vi "script - Copy.vi"() -> ()   [LabVIEW 2021]
panel:
  out "VI Name 2":string
  out "Application:All VIs In Memory 2":string[](array[string])
  out "VI Name":string
  out "appended array":errorcluster[](array[cluster])
  out "Application:All VIs In Memory":string[](array[string])
  out "error out":errorcluster
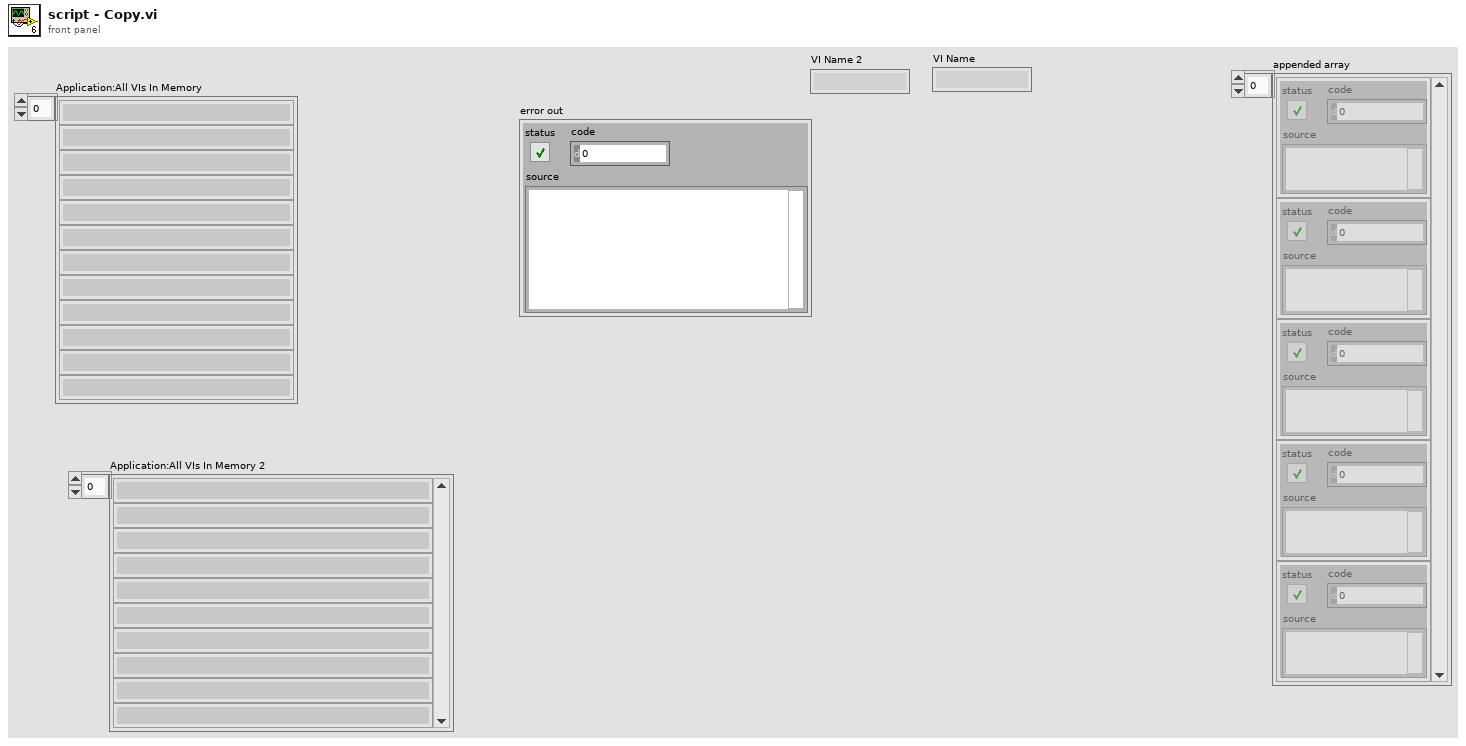
[diagram p1: front panel]
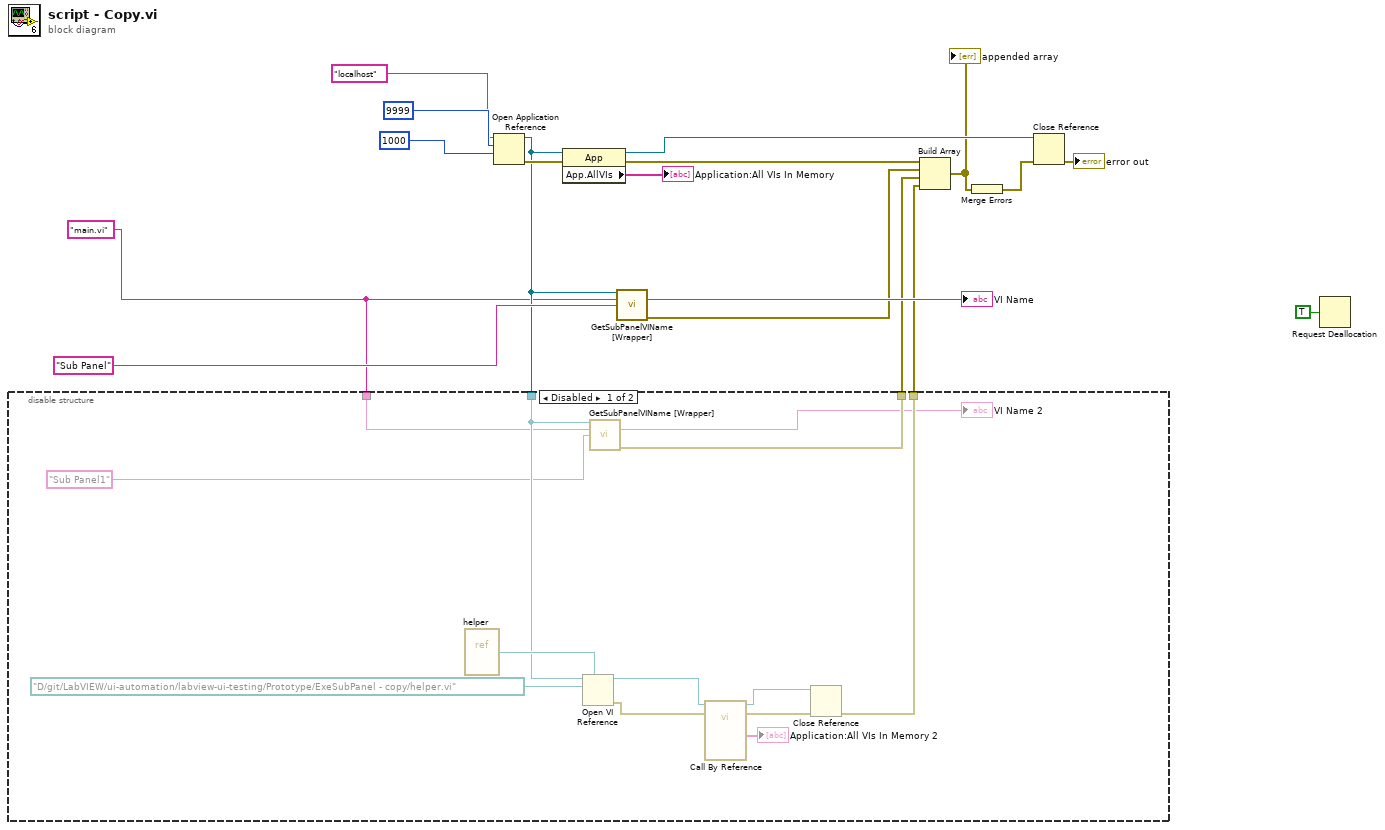
[diagram p0: block diagram]
diagram:
  w5 = "main.vi" ("y")
  n1 = Open Application Reference(9:1000 ("timeout ms (60000)"), 10:u16 9999 ("port number or service name (3363)"), 11:"localhost" ("machine name (\"\":  open local reference)")) -> (0:w17:errorcluster, 3:w6:refnum<vi>)  [unwired: 1 in]
  n2 = disable-structure shown="Disabled" {
    disable-tunnel: [w24 _] -> w8
    disable-tunnel: w6 -> [w23 _]
    disable-tunnel: w5 -> [w22 _]
    disable-tunnel: [w21 _] -> w4
    frame Disabled {
      n3 = vi-ref "helper.vi"() -> (w30:refnum<vi>)
      n4 = Open VI Reference(type specifier VI Refnum (for type only)=w30, application reference (local)=w23, vi path=path "D:/git/LabVIEW/ui-automation/labview-ui-testing/Prototype/ExeSubPanel - copy/helper.vi") -> (vi reference=w29:refnum<vi>, error out=w28:errorcluster)  [unwired: 3 in]
      n5 = call "GetSubPanelVIName [Wrapper].vi"("Application in"=w23, "VI Name"=w22, "SubPanel Label"="Sub Panel1" ("y")) -> ("VI Name"=→"VI Name 2":string, "error out"=w21:errorcluster)  [unwired: 10 in, 1 out]
      n6 = call-by-ref "?"(reference=w29, error in=w28) -> (reference out=w26:refnum<vi>, error out=w27:errorcluster, "Application:All VIs In Memory"=→"Application:All VIs In Memory 2":string[])  [unwired: 10 in, 1 out]
      n7 = Close Reference(reference=w26, error in (no error)=w27) -> (error out=w24:errorcluster)
    }
    frame Enabled {
    }
  }
  n8 = property class="App"(reference=w6, error in=w17) -> (reference out=w16:refnum<vi>, error out=w11:errorcluster, "App.AllVIs"=→"Application:All VIs In Memory":string[])
  n9 = call "GetSubPanelVIName [Wrapper].vi"("Application in"=w6, "VI Name"=w5, "SubPanel Label"="Sub Panel" ("y")) -> ("VI Name"=→"VI Name":string, "error out"=w7:errorcluster)  [unwired: 10 in, 1 out]
  n10 = Build Array(w11, w7, w4, w8) -> (w13:errorcluster[])
  "appended array" <- w13
  n11 = Merge Errors(w13) -> (w12:errorcluster)
  n12 = Close Reference(reference=w16, error in (no error)=w12) -> (error out=→"error out":errorcluster)
  n13 = Request Deallocation(TRUE ("flag")) -> ()
